vi "get status calb.vi"(8 "error in (no error)":errorcluster, 9 "calibration":cluster{"A":dbl, "MicrostepMode":u32}, 10 "status":T1, 11 "id":i32) -> (0 "error out":errorcluster, 2 "status out":T1, 3 "function return":i32)   [LabVIEW 2012, in "libximc.lvlib"]
doc: "result_t XIMC_API get_status_calb (device_t id, status_calb_t* status, const calibration_t* calibration);"
uses:
  libximc.lvlib
  libximc.dll
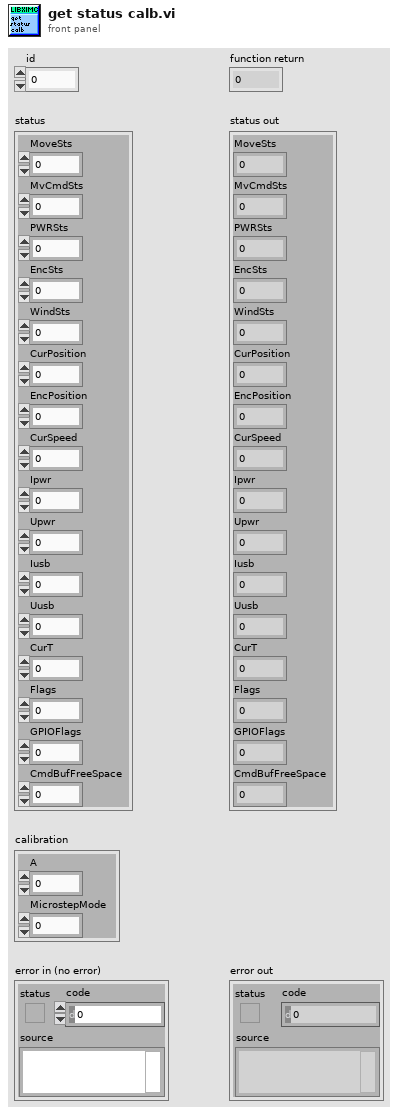
[diagram p1: front panel]
types:
  T1 = cluster{"MoveSts":u32, "MvCmdSts":u32, "PWRSts":u32, "EncSts":u32, "WindSts":u32, "CurPosition":sgl, "EncPosition":i64, "CurSpeed":sgl, "Ipwr":i32, "Upwr":i32, "Iusb":i32, "Uusb":i32, "CurT":i32, "Flags":u32, "GPIOFlags":u32, "CmdBufFreeSpace":u32}
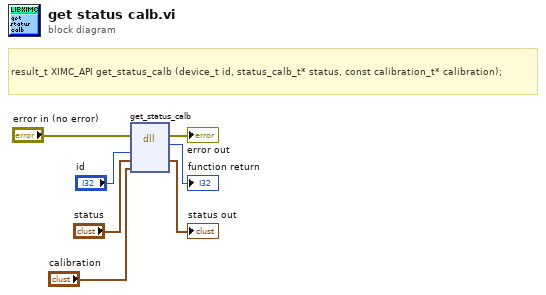
[diagram p0: block diagram]
diagram:
  # "result_t XIMC_API get_status_calb (device_t id, status_calb_t* status, const calibration_t* calibration);"
  n1 = dll-call lib="C:/Users/Stepan/Downloads/labview_2.9.11_testgen_thread/libximc.*" fn="get_status_calb"(error in="error in (no error)", "id"="id", "status"="status", "calibration"="calibration") -> (error out=→"error out":errorcluster, →"function return":i32, "status"=→"status out":T1)  [unwired: 4 in, 1 out]
